vi "function3.vi"(1 "y":dbl) -> (0 "x+y":dbl)   [LabVIEW 2012]
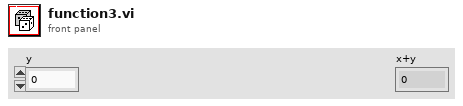
[diagram p1: front panel]
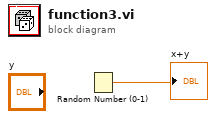
[diagram p0: block diagram]
diagram:
  n1 = Random Number (0-1)() -> (number: 0 to 1=→"x+y":dbl)
